vi "ACDC_Config_9234.vi"(8 "error in (no error)":errorcluster, 9 "Input Config Array":T1[](array[typedef])=[0, 0, 0, 0, 0, 0, 0, 0, 0, 0, 0, 0, 0, 0, 0, 0, 0, 0, 0, 0, 0, 0, 0, 0, 0, 0, 0, 0, 0, 0, 0, 0] items=["AC Coupled", "DC Coupled", "IEPE AC Coupled"], 10 "Data Rate [S/s]":u32) -> (0 "error out":errorcluster)   [LabVIEW 2017, in "BOP_VibAPI_8.lvlib"]
uses:
  <vilib>/addons/InsightCM/Devices/Shared/Cms/Fpga/Acquisition/source/subVIs/VibAPI_8/BOP_VibAPI_8.lvlib
  <vilib>/LabVIEW Targets/FPGA/cRIO/shared/nicrio_ModuleControls/nicrio_cRIO-9232_ConfigModeRing.ctl
  <vilib>/rvi/eio/common/nirviEmuTemplatePropertySet_errors.vi
  <vilib>/eio/EIOPropertyNode/EIOPropertyNode.xnode
  <vilib>/LabVIEW Targets/FPGA/cRIO/shared/nicrio_ModuleControls/nicrio_cRIO-9234_DataRatesRing2.ctl
  <vilib>/LabVIEW Targets/FPGA/cRIO/shared/nicrio_ModuleControls/nicrio_cRIO-9234_ConfigModeRing.ctl
  <vilib>/rvi/eio/common/nirviEmuTemplatePropertyGet_errors.vi
  <vilib>/rvi/eio/common/nirviEmuTemplatePropertyGet_noerrors.vi
  <vilib>/rvi/eio/common/nirviEmuTemplatePropertySet_noerrors.vi
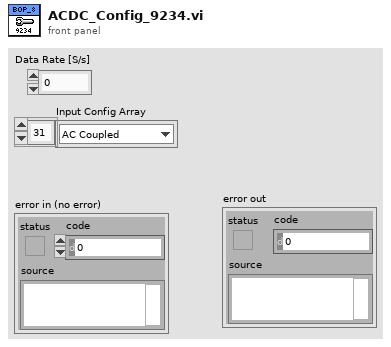
[diagram p1: front panel]
types:
  T1 = typedef "nicrio_cRIO-9232_ConfigModeRing.ctl" = u8
  T2 = typedef "nicrio_cRIO-9234_DataRatesRing2.ctl" = u8
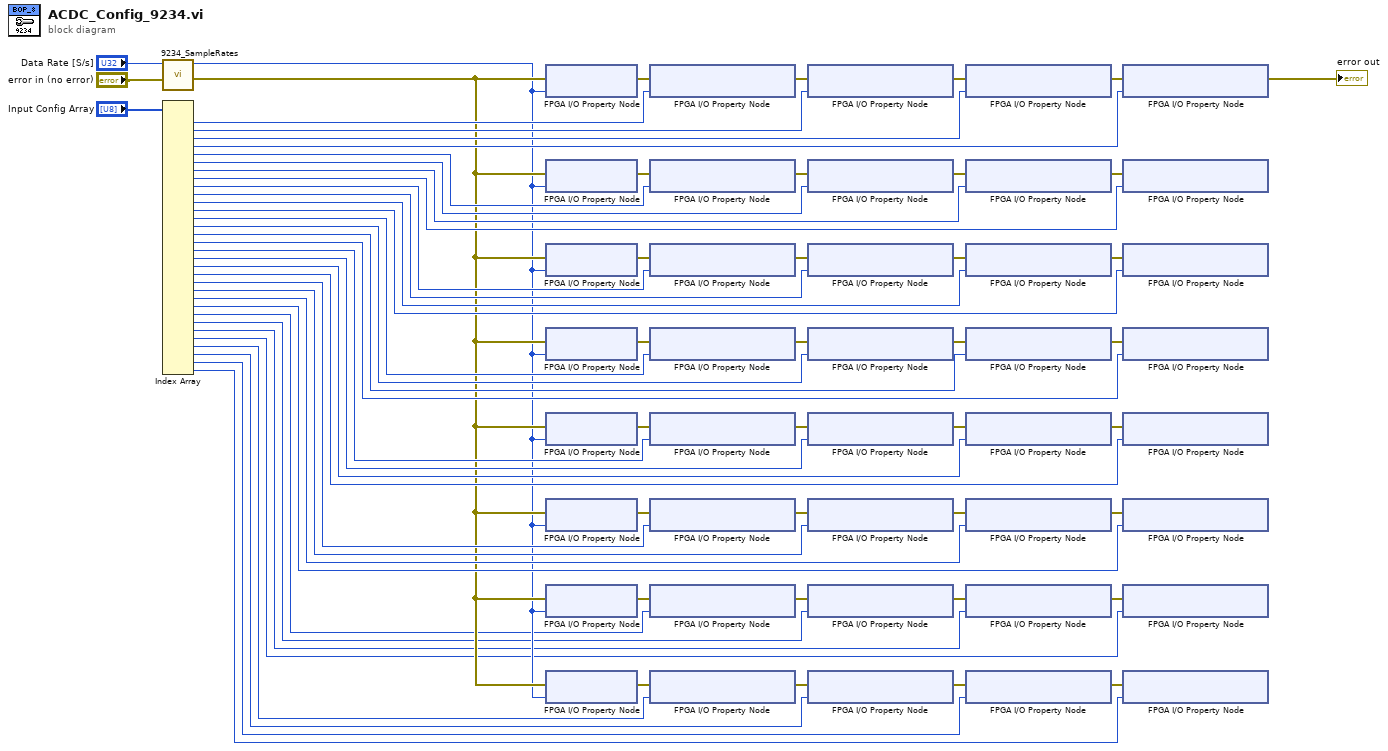
[diagram p0: block diagram]
diagram:
  n1 = call <vilib>:"9234_SampleRates.vi"("error in (no error)"="error in (no error)", "Data Rate [S/s]"="Data Rate [S/s]") -> ("error out"=w10:errorcluster, "Data Rate"=w9:T2)  [unwired: 8 in]
  n2 = Index Array(array="Input Config Array") -> (element #1=w27:T1, element #2=w28:T1, element #3=w29:T1, element #4=w68:T1, element #5=w67:T1, element #6=w66:T1, element #7=w65:T1, element #8=w64:T1, element #9=w63:T1, element #10=w62:T1, element #11=w61:T1, element #12=w60:T1, element #13=w59:T1, element #14=w58:T1, element #15=w57:T1, element #16=w56:T1, element #17=w55:T1, element #18=w54:T1, element #19=w53:T1, element #20=w52:T1, element #21=w51:T1, element #22=w50:T1, element #23=w49:T1, element #24=w48:T1, element #25=w8:T1, element #26=w7:T1, element #27=w6:T1, element #28=w5:T1, element #29=w4:T1, element #30=w3:T1, element #31=w2:T1, element #32=w1:T1)  [unwired: 32 in]
  n3 = xnode "FPGA I/O Property Node"("error in"=w10, "Data Rate"=w9) -> ("error out"=w25:errorcluster)  [unwired: 1 in, 1 out]
  n4 = xnode "FPGA I/O Property Node"("error in"=w10, "Data Rate"=w9) -> ("error out"=w26:errorcluster)  [unwired: 1 in, 1 out]
  n5 = xnode "FPGA I/O Property Node"("error in"=w10, "Data Rate"=w9) -> ("error out"=w30:errorcluster)  [unwired: 1 in, 1 out]
  n6 = xnode "FPGA I/O Property Node"("error in"=w10, "Data Rate"=w9) -> ("error out"=w35:errorcluster)  [unwired: 1 in, 1 out]
  n7 = xnode "FPGA I/O Property Node"("error in"=w10, "Data Rate"=w9) -> ("error out"=w36:errorcluster)  [unwired: 1 in, 1 out]
  n8 = xnode "FPGA I/O Property Node"("error in"=w10, "Data Rate"=w9) -> ("error out"=w41:errorcluster)  [unwired: 1 in, 1 out]
  n9 = xnode "FPGA I/O Property Node"("error in"=w10, "Data Rate"=w9) -> ("error out"=w18:errorcluster)  [unwired: 1 in, 1 out]
  n10 = xnode "FPGA I/O Property Node"("error in"=w10, "Data Rate"=w9) -> ("error out"=w13:errorcluster)  [unwired: 1 in, 1 out]
  n11 = xnode "FPGA I/O Property Node"("error in"=w25, "Input Configuration"=w27) -> ("error out"=w24:errorcluster)  [unwired: 1 in, 1 out]
  n12 = xnode "FPGA I/O Property Node"("error in"=w26, "Input Configuration"=w67) -> ("error out"=w22:errorcluster)  [unwired: 1 in, 1 out]
  n13 = xnode "FPGA I/O Property Node"("error in"=w30, "Input Configuration"=w63) -> ("error out"=w31:errorcluster)  [unwired: 1 in, 1 out]
  n14 = xnode "FPGA I/O Property Node"("error in"=w35, "Input Configuration"=w59) -> ("error out"=w34:errorcluster)  [unwired: 1 in, 1 out]
  n15 = xnode "FPGA I/O Property Node"("error in"=w36, "Input Configuration"=w55) -> ("error out"=w37:errorcluster)  [unwired: 1 in, 1 out]
  n16 = xnode "FPGA I/O Property Node"("error in"=w41, "Input Configuration"=w51) -> ("error out"=w40:errorcluster)  [unwired: 1 in, 1 out]
  n17 = xnode "FPGA I/O Property Node"("error in"=w18, "Input Configuration"=w8) -> ("error out"=w17:errorcluster)  [unwired: 1 in, 1 out]
  n18 = xnode "FPGA I/O Property Node"("error in"=w13, "Input Configuration"=w4) -> ("error out"=w14:errorcluster)  [unwired: 1 in, 1 out]
  n19 = xnode "FPGA I/O Property Node"("error in"=w24, "Input Configuration"=w28) -> ("error out"=w23:errorcluster)  [unwired: 1 in, 1 out]
  n20 = xnode "FPGA I/O Property Node"("error in"=w22, "Input Configuration"=w66) -> ("error out"=w21:errorcluster)  [unwired: 1 in, 1 out]
  n21 = xnode "FPGA I/O Property Node"("error in"=w31, "Input Configuration"=w62) -> ("error out"=w32:errorcluster)  [unwired: 1 in, 1 out]
  n22 = xnode "FPGA I/O Property Node"("error in"=w34, "Input Configuration"=w58) -> ("error out"=w33:errorcluster)  [unwired: 1 in, 1 out]
  n23 = xnode "FPGA I/O Property Node"("error in"=w37, "Input Configuration"=w54) -> ("error out"=w38:errorcluster)  [unwired: 1 in, 1 out]
  n24 = xnode "FPGA I/O Property Node"("error in"=w40, "Input Configuration"=w50) -> ("error out"=w39:errorcluster)  [unwired: 1 in, 1 out]
  n25 = xnode "FPGA I/O Property Node"("error in"=w17, "Input Configuration"=w7) -> ("error out"=w16:errorcluster)  [unwired: 1 in, 1 out]
  n26 = xnode "FPGA I/O Property Node"("error in"=w14, "Input Configuration"=w3) -> ("error out"=w15:errorcluster)  [unwired: 1 in, 1 out]
  n27 = xnode "FPGA I/O Property Node"("error in"=w23, "Input Configuration"=w29) -> ("error out"=w42:errorcluster)  [unwired: 1 in, 1 out]
  n28 = xnode "FPGA I/O Property Node"("error in"=w21, "Input Configuration"=w65) -> ("error out"=w43:errorcluster)  [unwired: 1 in, 1 out]
  n29 = xnode "FPGA I/O Property Node"("error in"=w32, "Input Configuration"=w61) -> ("error out"=w44:errorcluster)  [unwired: 1 in, 1 out]
  n30 = xnode "FPGA I/O Property Node"("error in"=w33, "Input Configuration"=w57) -> ("error out"=w45:errorcluster)  [unwired: 1 in, 1 out]
  n31 = xnode "FPGA I/O Property Node"("error in"=w38, "Input Configuration"=w53) -> ("error out"=w46:errorcluster)  [unwired: 1 in, 1 out]
  n32 = xnode "FPGA I/O Property Node"("error in"=w39, "Input Configuration"=w49) -> ("error out"=w47:errorcluster)  [unwired: 1 in, 1 out]
  n33 = xnode "FPGA I/O Property Node"("error in"=w16, "Input Configuration"=w6) -> ("error out"=w12:errorcluster)  [unwired: 1 in, 1 out]
  n34 = xnode "FPGA I/O Property Node"("error in"=w15, "Input Configuration"=w2) -> ("error out"=w11:errorcluster)  [unwired: 1 in, 1 out]
  n35 = xnode "FPGA I/O Property Node"("error in"=w42, "Input Configuration"=w68) -> ("error out"=→"error out":errorcluster)  [unwired: 1 in, 1 out]
  n36 = xnode "FPGA I/O Property Node"("error in"=w43, "Input Configuration"=w64) -> ()  [unwired: 1 in, 2 out]
  n37 = xnode "FPGA I/O Property Node"("error in"=w44, "Input Configuration"=w60) -> ()  [unwired: 1 in, 2 out]
  n38 = xnode "FPGA I/O Property Node"("error in"=w45, "Input Configuration"=w56) -> ()  [unwired: 1 in, 2 out]
  n39 = xnode "FPGA I/O Property Node"("error in"=w46, "Input Configuration"=w52) -> ()  [unwired: 1 in, 2 out]
  n40 = xnode "FPGA I/O Property Node"("error in"=w47, "Input Configuration"=w48) -> ()  [unwired: 1 in, 2 out]
  n41 = xnode "FPGA I/O Property Node"("error in"=w12, "Input Configuration"=w5) -> ()  [unwired: 1 in, 2 out]
  n42 = xnode "FPGA I/O Property Node"("error in"=w11, "Input Configuration"=w1) -> ()  [unwired: 1 in, 2 out]
